vi "parse device list by type.vi"(2 "DeviceListin":T1(array[cluster])) -> (0 "DeviceListout":T1(array[cluster]))   [LabVIEW 2013]
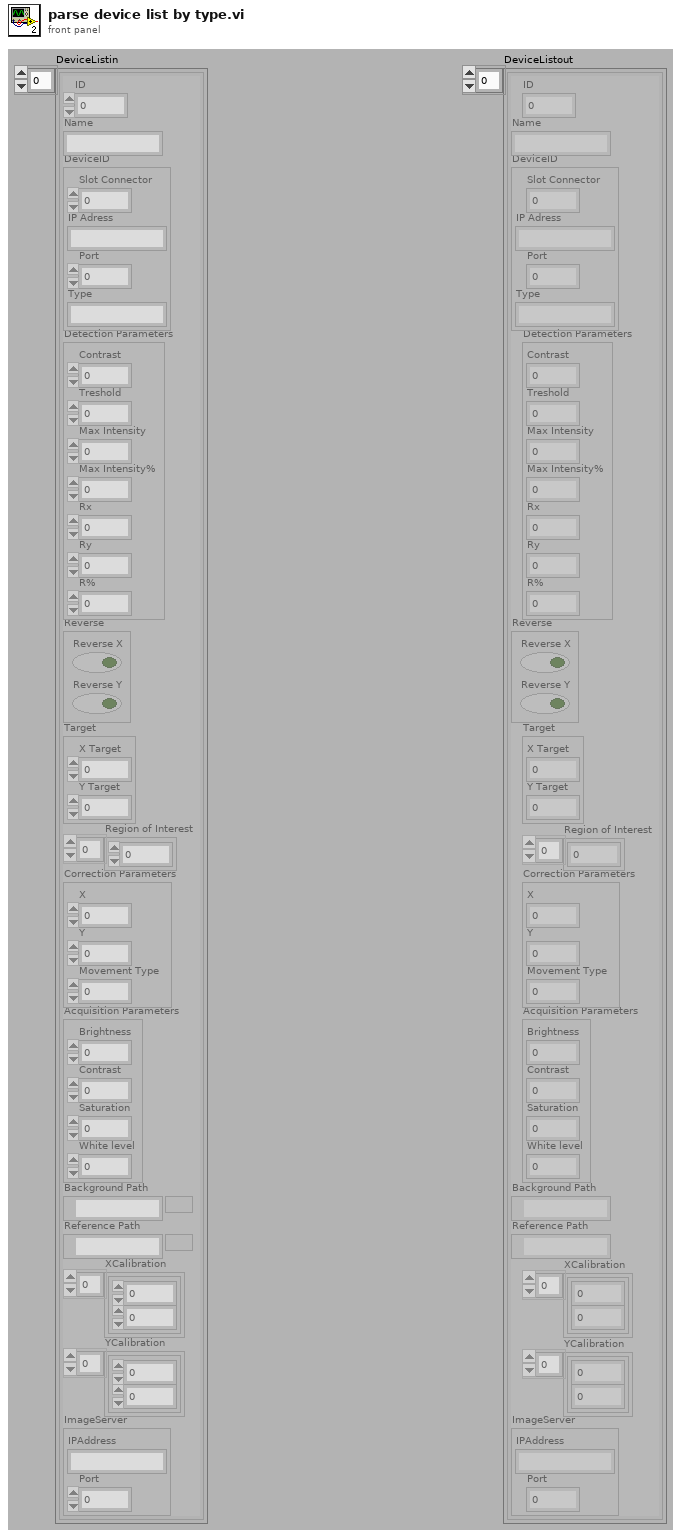
[diagram p1: front panel]
types:
  T1 = cluster{"ID":dbl, "Name":string, "DeviceID":cluster{"Slot Connector":i32, "IP Adress":string, "Port":i32, "Type":string}, "Detection Parameters":cluster{"Contrast":i32, "Treshold":u8, "Max Intensity":i32, "Max Intensity%":u8, "Rx":i32, "Ry":i32, "R%":sgl}, "Reverse":cluster{"Reverse X":bool, "Reverse Y":bool}, "Target":cluster{"X Target":sgl, "Y Target":sgl}, "Region of Interest":i32[], "Correction Parameters":cluster{"X":sgl, "Y":sgl, "Movement Type":u16}, "Acquisition Parameters":cluster{"Brightness":dbl, "Contrast":dbl, "Saturation":dbl, "White level":dbl}, "Background Path":path, "Reference Path":path, "XCalibration":cluster{dbl, dbl}[], "YCalibration":cluster{dbl, dbl}[], "ImageServer":cluster{"IPAddress":string, "Port":i32}}[]
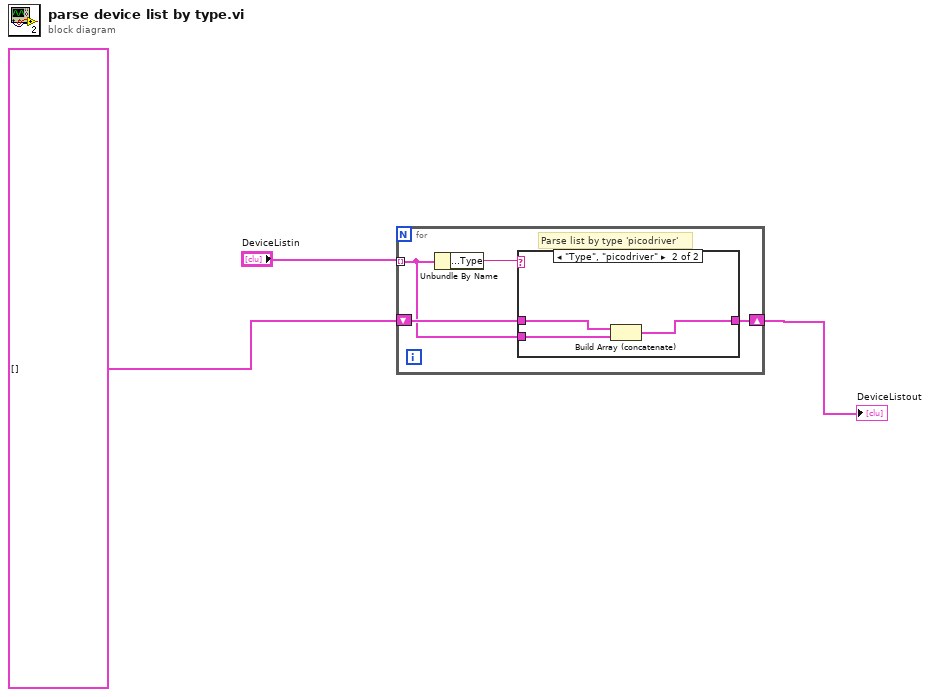
[diagram p0: block diagram]
diagram:
  n1 = for {
    tunnel: "DeviceListin" -> [w5] mode=indexing
    shift-right: [w7] -> w2
    shift-left: T1 [] ("EmptyDeviceList") -> [w6]
    # "Parse list by type 'picodriver'"
    n2 = Unbundle By Name(w5) -> ("DeviceID.Type"=w4:string)
    n3 = case shown="\"Type\", \"picodriver\"" w4 {
      tunnel: w5 -> [_ w11]
      tunnel: [w8 w10] -> w7
      tunnel: w6 -> [w8 w9]
      frame "False", Default {
      }
      frame "Type", "picodriver" {
        n4 = Build Array (concatenate)(w9, w11) -> (w10:T1)
      }
    }
  }
  "DeviceListout" <- w2
